vi "通讯标准化.vi"() -> ()   [LabVIEW 2018]
uses:
  <vilib>/Instr/_visa.llb/VISA Configure Serial Port (Instr).vi
panel:
  in  "写入命令":string
  out "通讯数据":string
  in  "协议状态":bool
  in  "串口配置参数":T1={"VISA resource name"="", "baud rate (9600)"=9600, "data bits (8)"=8, "parity (0:none)"=enum."None", "stop bits (10: 1 bit)"=10, "timeout (10sec)"=10000, "Enable Termination\nChar (T)"=TRUE, "termination char\n(0xA = '\\n' = LF) "=10, "flow control (0:none)"=0} {"flow control (0:none)" items=["无", "XON/XOFF", "RTS/CTS", "XON/XOFF & RTS/CTS", "DTR/DSR", "XON/XOFF & DTR/DSR"]; "termination char\n(0xA = '\\n' = LF)" format="%.0x"; "stop bits (10: 1 bit)" items=["1.0"=10, "1.5"=15, "2.0"=20]; "data bits (8)" min=5 max=8 step=1}
  in  "操作方式":enum16{"只读", "只写", "读/写"}(ring)
  in  "通讯方式":enum16{"串口", "以太网"}(ring)
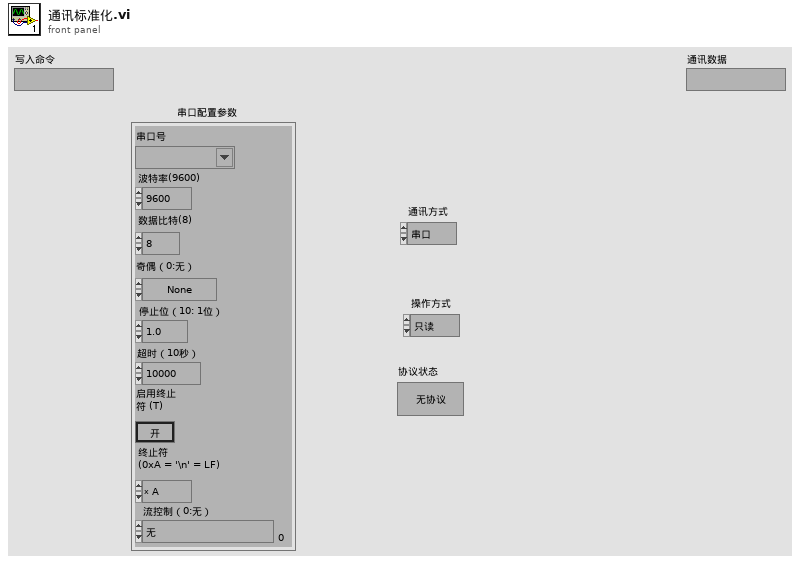
[diagram p1: front panel]
types:
  T1 = cluster{"VISA resource name":refnum<visa-resource-name>, "baud rate (9600)":u32, "data bits (8)":u16, "parity (0:none)":enum16{"None", "Odd", "Even", "Mark", "Space"}, "stop bits (10: 1 bit)":u16, "timeout (10sec)":u32, "Enable Termination\nChar (T)":bool, "termination char\n(0xA = '\\n' = LF) ":u8, "flow control (0:none)":u16}
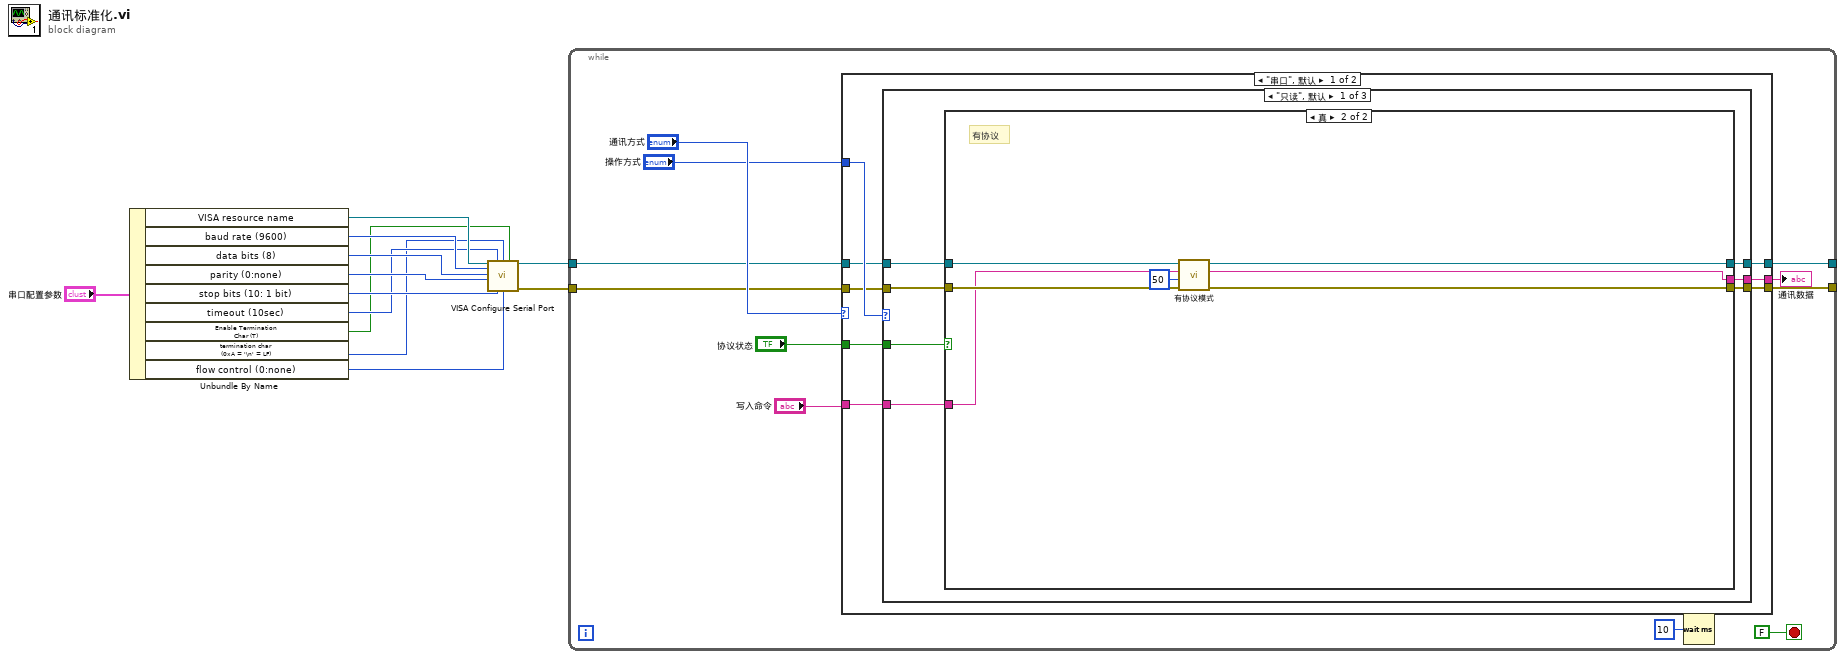
[diagram p0: block diagram]
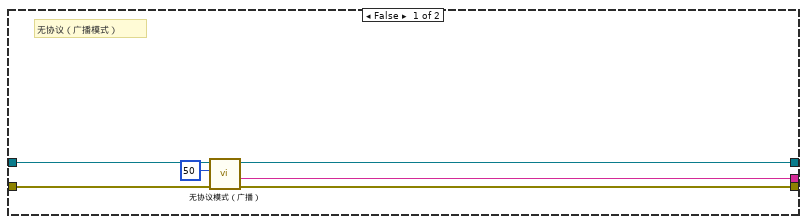
[diagram p2: hidden frame]
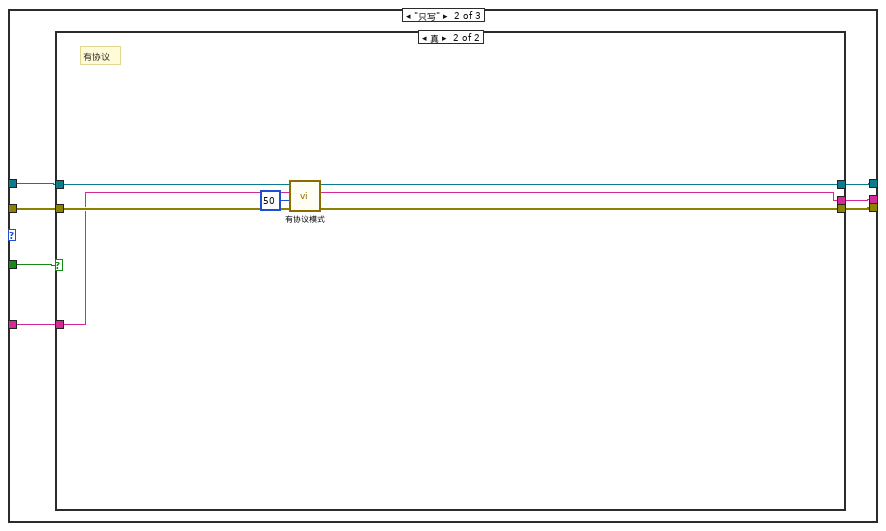
[diagram p3: hidden frame]
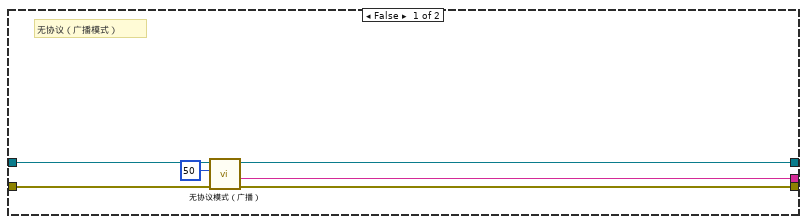
[diagram p4: hidden frame]
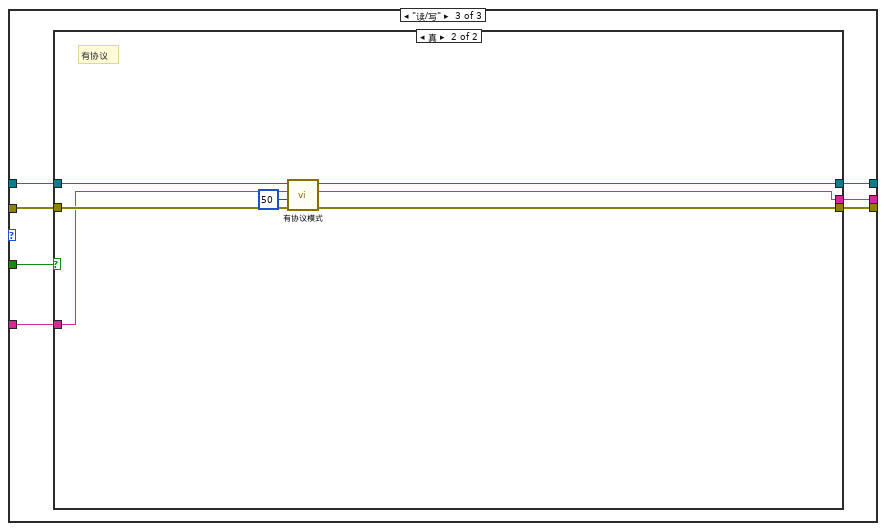
[diagram p5: hidden frame]
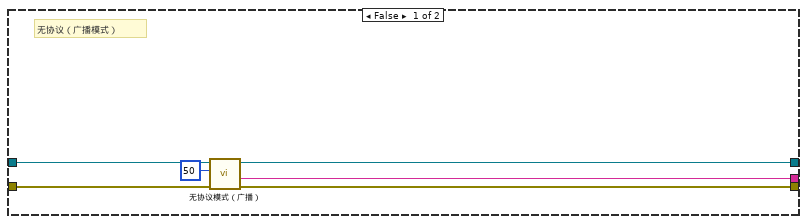
[diagram p6: hidden frame]
diagram:
  n1 = Unbundle By Name("串口配置参数") -> ("VISA resource name"=w9:refnum<visa-resource-name>, "baud rate (9600)"=w8:u32, "data bits (8)"=w7:u16, "parity (0:none)"=w6:enum16{"None", "Odd", "Even", "Mark", "Space"}, "stop bits (10: 1 bit)"=w5:u16, "timeout (10sec)"=w4:u32, "Enable Termination\nChar (T)"=w1:bool, "termination char\n(0xA = '\\n' = LF)"=w2:u8, "flow control (0:none)"=w3:u16)
  n2 = call-poly "VISA Configure Serial Port"("VISA resource name"=w9, "timeout (10sec)"=w4, "termination char\n(0xA = '\\n' = LF)"=w2, "Enable Termination\nChar (T)"=w1, "baud rate (9600)"=w8, "data bits (8)"=w7, "parity (0:none)"=w6, "stop bits (10: 1 bit)"=w5, "flow control (0:none)"=w3) -> ("VISA resource name out"=w12:refnum<visa-resource-name>, "error out"=w11:errorcluster)  [unwired: 5 in]
  n3 = while {
    tunnel: w12 -> [w21]
    tunnel: w11 -> [w20]
    tunnel: [w17] -> _
    tunnel: [w16] -> _
    stop <- FALSE stop-if-true
    n4 = case shown="\"串口\", 默认" "通讯方式" {
      tunnel: "操作方式" -> [w31 w92]
      tunnel: w21 -> [w30 _]
      tunnel: w20 -> [w29 _]
      tunnel: "协议状态" -> [w28 _]
      tunnel: [w27 _] -> w17
      tunnel: [w26 _] -> w16
      tunnel: [w25 _] -> w14
      tunnel: "写入命令" -> [w24 _]
      frame "串口", Default {
        n5 = case shown="\"只读\", 默认" w31 {
          tunnel: w30 -> [w37 w58 w78]
          tunnel: w29 -> [w36 w57 w77]
          tunnel: w28 -> [w38 w56 w73]
          tunnel: [w35 w55 w76] -> w27
          tunnel: [w34 w54 w75] -> w26
          tunnel: [w33 w53 w74] -> w25
          tunnel: w24 -> [w32 w52 w72]
          frame "只读", Default {
            n6 = case shown="真" w38 {
              tunnel: w37 -> [w44 w51]
              tunnel: w36 -> [w42 w50]
              tunnel: [w43 w48] -> w35
              tunnel: [w41 w47] -> w34
              tunnel: [w39 w46] -> w33
              tunnel: w32 -> [_ w45]
              frame False {
                # "无协议（广播模式）"
                n7 = call "无协议模式（广播）.vi"("错误输入（无错误）"=w42, "等待时间（毫秒）"=u32 50, "VISA资源名称"=w44) -> ("错误输出"=w41:errorcluster, "通讯数据"=w39:string, "VISA资源名称输出"=w43:refnum<visa-resource-name>)  [unwired: 6 in]
              }
              frame True {
                # "有协议"
                n8 = call "有协议模式.vi"("错误输入（无错误）"=w50, "等待时间"=u32 50, "写入命令"=w45, "VISA资源名称"=w51) -> ("错误输出"=w47:errorcluster, "通讯数据"=w46:string, "VISA资源名称输出"=w48:refnum<visa-resource-name>)  [unwired: 5 in]
              }
            }
          }
          frame "只写" {
            n9 = case shown="真" w56 {
              tunnel: w58 -> [w64 w71]
              tunnel: w57 -> [w62 w70]
              tunnel: [w63 w68] -> w55
              tunnel: [w61 w67] -> w54
              tunnel: [w59 w66] -> w53
              tunnel: w52 -> [_ w65]
              frame False {
                # "无协议（广播模式）"
                n10 = call "无协议模式（广播）.vi"("错误输入（无错误）"=w62, "等待时间（毫秒）"=u32 50, "VISA资源名称"=w64) -> ("错误输出"=w61:errorcluster, "通讯数据"=w59:string, "VISA资源名称输出"=w63:refnum<visa-resource-name>)  [unwired: 6 in]
              }
              frame True {
                # "有协议"
                n11 = call "有协议模式.vi"("错误输入（无错误）"=w70, "等待时间"=u32 50, "写入命令"=w65, "VISA资源名称"=w71) -> ("错误输出"=w67:errorcluster, "通讯数据"=w66:string, "VISA资源名称输出"=w68:refnum<visa-resource-name>)  [unwired: 5 in]
              }
            }
          }
          frame "读/写" {
            n12 = case shown="真" w73 {
              tunnel: w78 -> [w84 w91]
              tunnel: w77 -> [w82 w90]
              tunnel: [w83 w88] -> w76
              tunnel: [w81 w87] -> w75
              tunnel: [w79 w86] -> w74
              tunnel: w72 -> [_ w85]
              frame False {
                # "无协议（广播模式）"
                n13 = call "无协议模式（广播）.vi"("错误输入（无错误）"=w82, "等待时间（毫秒）"=u32 50, "VISA资源名称"=w84) -> ("错误输出"=w81:errorcluster, "通讯数据"=w79:string, "VISA资源名称输出"=w83:refnum<visa-resource-name>)  [unwired: 6 in]
              }
              frame True {
                # "有协议"
                n14 = call "有协议模式.vi"("错误输入（无错误）"=w90, "等待时间"=u32 50, "写入命令"=w85, "VISA资源名称"=w91) -> ("错误输出"=w87:errorcluster, "通讯数据"=w86:string, "VISA资源名称输出"=w88:refnum<visa-resource-name>)  [unwired: 5 in]
              }
            }
          }
        }
      }
      frame "以太网" {
        n15 = case shown="\"只读\", 默认" w92 {
          frame "只读", Default {
          }
          frame "只写" {
          }
          frame "读/写" {
          }
        }
      }
    }
    "通讯数据" <- w14
    n16 = Wait (ms)(milliseconds to wait=u32 10 ("等待时间（毫秒）")) -> ()  [unwired: 1 out]
  }
